vi "ntitled 2.vi"() -> ()   [LabVIEW 2020]
panel:
  out "Datos":dynamicdata(graph)
  in  "?":bool
  out "Alarma":bool
  out "Limite":dbl
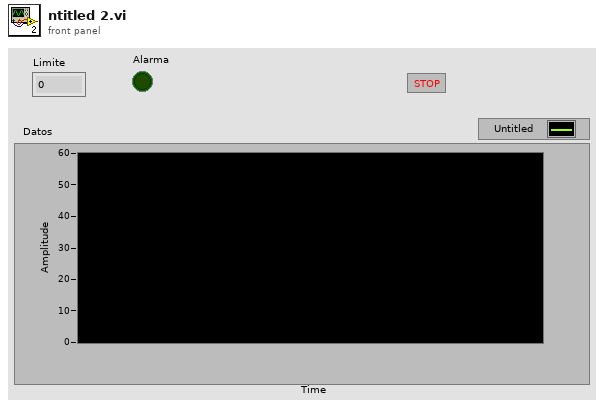
[diagram p1: front panel]
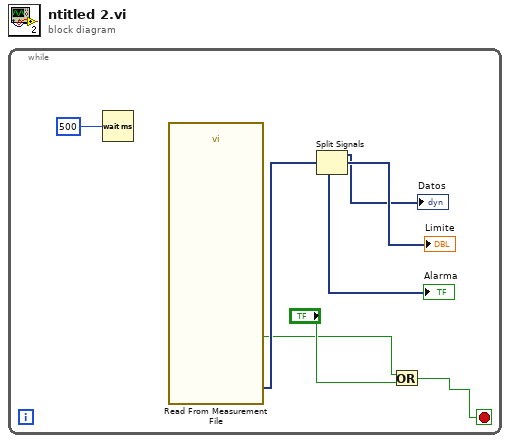
[diagram p0: block diagram]
diagram:
  n1 = while {
    stop <- w4 stop-if-true
    n2 = Wait (ms)(milliseconds to wait=500) -> ()  [unwired: 1 out]
    n3 = call "Read From Measurement File"() -> ("Signals"=w6:dynamicdata, "EOF?"=w1:bool)  [unwired: 6 in, 4 out]
    n4 = Split Signals "Split Signals"(w6) -> (→"Datos":dynamicdata, →"Limite":dynamicdata, →"Alarma":dynamicdata)  [unwired: 3 in]
    n5 = Or(x=w1, y="?") -> (x .or. y?=w4:bool)
  }
